vi "subIsInViLib.vi"(8 "error in (no error)":errorcluster, 11 "VI Refnum":refnum<vi>) -> (0 "error out":errorcluster, 2 "In vi.lib?":bool, 3 "dup VI Refnum":refnum<vi>)   [LabVIEW 2014, in "lvbuildsecurity.lvlib"]
uses:
  lvbuildsecurity.lvlib
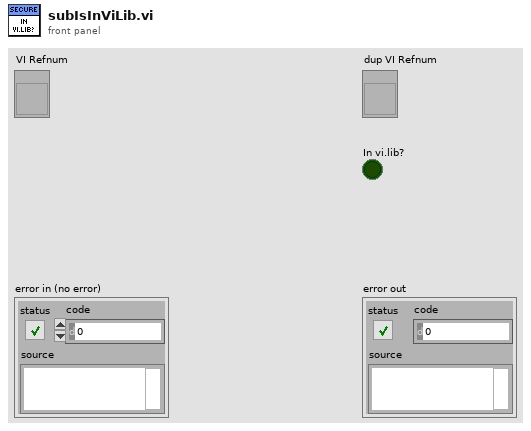
[diagram p1: front panel]
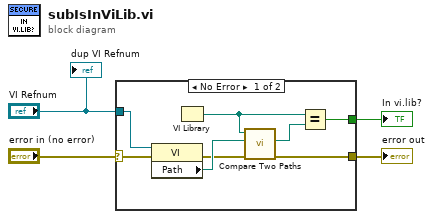
[diagram p0: block diagram]
diagram:
  n1 = case shown="No Error" "error in (no error)" {
    selector: "error in (no error)" -> [w8 w13]
    tunnel: "VI Refnum" -> [w7 _]
    tunnel: [w6 _] -> w1
    tunnel: [w5 w13] -> w2
    frame No Error {
      n2 = property class="VI"(reference=w7, error in=w8) -> (error out=w11:errorcluster, "Path"=w12:path)  [unwired: 1 out]
      n3 = VI Library() -> (path=w9:path)
      n4 = call <vilib>:"Compare Two Paths.vi"("error in (no error)"=w11, "Path 2"=w12, "Path 1"=w9) -> ("error out"=w5:errorcluster, "Common Path"=w10:path)  [unwired: 5 in, 2 out]
      n5 = Equal?(x=w9, y=w10) -> (x = y?=w6:bool)
    }
    frame Error {
    }
  }
  "error out" <- w2
  "In vi.lib?" <- w1
  "dup VI Refnum" <- "VI Refnum"
